vi "GetSpeedProperties.vi"(10 "Channels":T1[](array[typedef]), 11 "properties":T2[](array[typedef])) -> (1 "speed reference id":string, 2 "nominal speed":dbl, 3 "speed type":T4, 5 "max empty blocks":i32)   [LabVIEW 2017, in "AnalysisHelper.lvlib"]
uses:
  <vilib>/addons/InsightCM/Utilities/Analysis/Shared/AnalysisHelper.lvlib
  <vilib>/addons/InsightCM/MessageBus/Base/controls/KeyValuePair.ctl
  <vilib>/addons/InsightCM/Utilities/Analysis/Shared/controls/SpeedType.ctl
  <vilib>/addons/InsightCM/MessageBus/Base/controls/R2_Channel.ctl
  <vilib>/addons/InsightCM/MessageBus/Base/controls/Metric.ctl
  <vilib>/addons/InsightCM/Utilities/PropertyHelpers/PropertyHelpers.lvlib
  <vilib>/addons/InsightCM/Utilities/DeviceModelHelpers/DeviceModelHelpers.lvlib
  <vilib>/addons/InsightCM/Utilities/GlobalConfiguration/GlobalConfiguration.lvlib
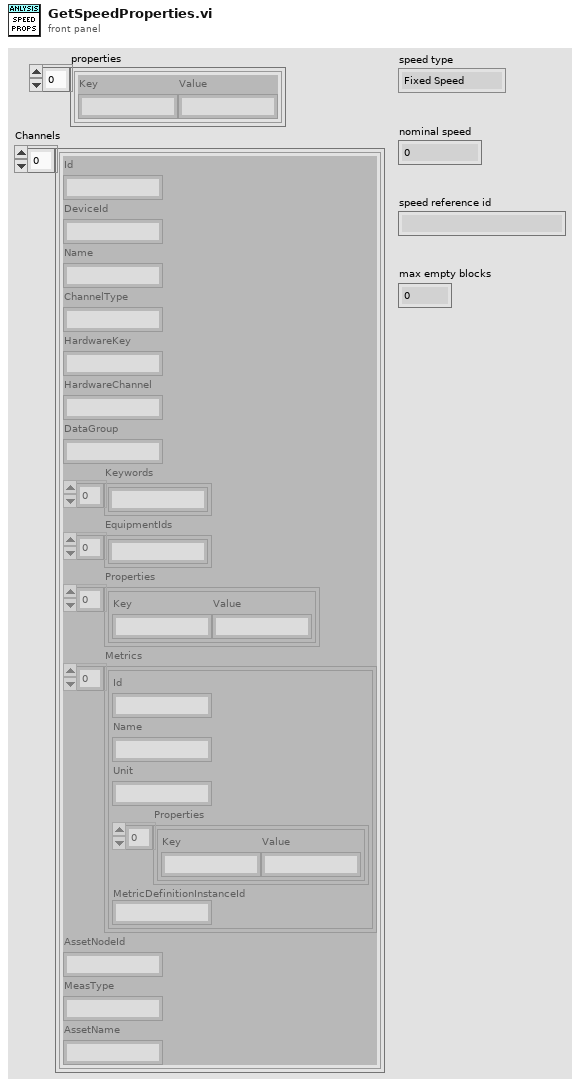
[diagram p1: front panel]
types:
  T1 = typedef "R2_Channel.ctl" = cluster{"Id":string, "DeviceId":string, "Name":string, "ChannelType":string, "HardwareKey":string, "HardwareChannel":string, "DataGroup":string, "Keywords":string[], "EquipmentIds":string[], "Properties":T2[], "Metrics":T3[], "AssetNodeId":string, "MeasType":string, "AssetName":string}
  T2 = typedef "KeyValuePair.ctl" = cluster{"Key":string, "Value":string}
  T3 = typedef "Metric.ctl" = cluster{"Id":string, "Name":string, "Unit":string, "Properties":T2[], "MetricDefinitionInstanceId":string}
  T4 = typedef "AnalysisHelper.lvlib/SpeedType.ctl" = enum16{"Fixed Speed", "Tachometer", "From Map"}
  T5 = typedef "SectionKeyValues.ctl" = cluster{"Section":string, "KeyValues":T2[]}
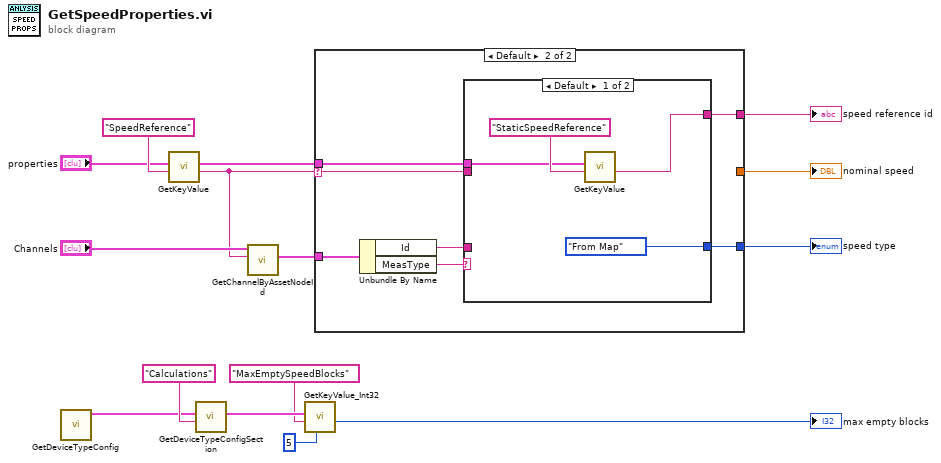
[diagram p0: block diagram]
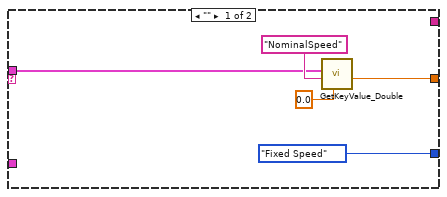
[diagram p2: hidden frame]
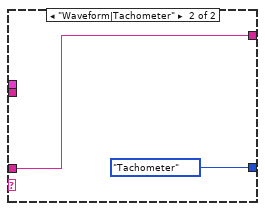
[diagram p3: hidden frame]
diagram:
  n1 = call <vilib>:"GetDeviceTypeConfig.vi"() -> ("key values"=w3:T5[])  [unwired: 9 in, 2 out]
  n2 = call <vilib>:"GetKeyValue.vi"("key"="SpeedReference", "key value pairs"="properties") -> ("value"=w8:string, "key value pairs out"=w12:T2[])  [unwired: 7 in, 1 out]
  n3 = call <vilib>:"GetDeviceTypeConfigSection.vi"("key"="Calculations", "key values"=w3) -> ("key value pairs out"=w5:T2[])  [unwired: 8 in, 1 out]
  n4 = call <vilib>:"GetChannelByAssetNodeId.vi"("channel id"=w8, "channels in"="Channels") -> ("channel"=w7:T1)  [unwired: 7 in, 2 out]
  n5 = call <vilib>:"GetKeyValue_Int32.vi"("default"=5, "key"="MaxEmptySpeedBlocks", "key value pairs"=w5) -> ("value"=→"max empty blocks":i32)  [unwired: 6 in, 2 out]
  n6 = case shown="Default" w8 {
    selector: w8 -> [_ w22]
    tunnel: w12 -> [w16 w24]
    tunnel: [SpeedType."Fixed Speed" ("Speed Type") w27] -> w15
    tunnel: [w17 _] -> w14
    tunnel: w7 -> [_ w26]
    tunnel: [_ w23] -> w10
    frame "" {
      n7 = call <vilib>:"GetKeyValue_Double.vi"("default"=0.0, "key"="NominalSpeed", "key value pairs"=w16) -> ("value"=w17:dbl)  [unwired: 6 in, 2 out]
    }
    frame Default {
      n8 = Unbundle By Name(w26) -> ("Id"=w21:string, "MeasType"=w25:string)
      n9 = case shown="Default" w25 {
        tunnel: [SpeedType."From Map" ("Speed Type") SpeedType."Tachometer" ("Speed Type")] -> w27
        tunnel: w24 -> [w29 _]
        tunnel: [w28 w32] -> w23
        tunnel: w22 -> [_ _]
        tunnel: w21 -> [_ w32]
        frame Default {
          n10 = call <vilib>:"GetKeyValue.vi"("key"="StaticSpeedReference", "key value pairs"=w29) -> ("value"=w28:string)  [unwired: 7 in, 2 out]
        }
        frame "Waveform|Tachometer" {
        }
      }
    }
  }
  "nominal speed" <- w14
  "speed reference id" <- w10
  "speed type" <- w15
